vi "Measurement_Param_Global_Var.vi"() -> ()   [LabVIEW 2017]
panel:
  out "Sweep Parameters":T1
  in  "Average_en":bool
  out "ADC Cnfg Data":T2
  in  "Iterations":u16=13 caption="Iterations per Step" step=1
  in  "Settling time":u32=13 caption="Settling Time (ms)" max=4095 step=1
  in  "Vcm_2":dbl caption="Vcm ADC_2 (V)" min=0.0 max=3.3 step=0.001 format="%#.3f"
  in  "Vcm_1":dbl caption="Vcm ADC_1 (V)" min=0.0 max=3.3 step=0.001 format="%#.3f"
  in  "Sweep Vref2":bool caption="Sweep"
  in  "Nb of steps Vref2":u16 caption="Nb of steps" max=4095 step=1
  in  "Step size Vref2":u16 caption="Step size" max=4095 step=1
  in  "ADC Vref2":u16 caption="Start Value" max=4095 step=1
  in  "Sweep Vref1":bool caption="Sweep"
  in  "Sweep Vin":bool caption="Sweep"
  in  "Nb of steps Vref1":u16 caption="Nb of steps" max=4095 step=1
  in  "Step size Vref1":u16 caption="Step size" max=4095 step=1
  in  "ADC Vref1":u16 caption="Start Value" max=4095 step=1
  in  "Nb of steps Vin":u16 caption="Nb of steps" step=1
  in  "Step size Vin":u16 caption="Step size" step=1
  in  "ADC Vin":u16 caption="Start Value" step=1
  # "ADC Vin"
  # "Vref ADC_1"
  # "Vref ADC_2"
  # "Vcm"
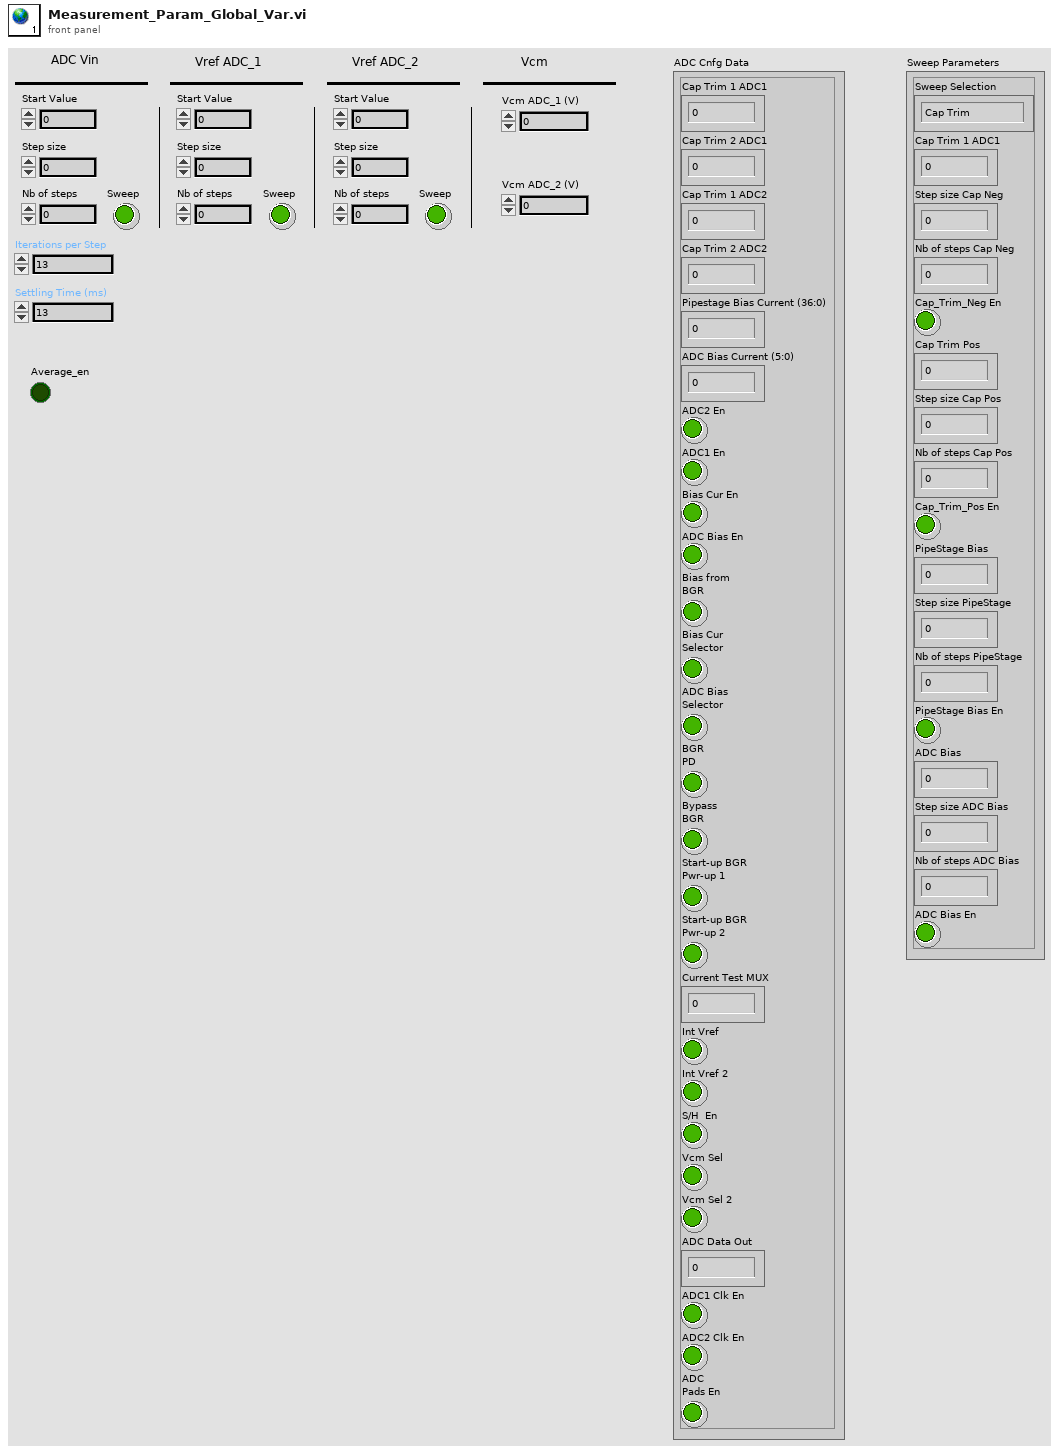
[diagram p1: front panel]
types:
  T1 = cluster{"Sweep Selection":enum32{"Cap Trim", "Bias Current", "Vreference"}, "Cap Trim 1 ADC1":u16, "Step size Cap Neg":u16, "Nb of steps Cap Neg":u16, "Cap_Trim_Neg En":bool, "Cap Trim Pos":u16, "Step size Cap Pos":u16, "Nb of steps Cap Pos":u16, "Cap_Trim_Pos En":bool, "PipeStage Bias":u64, "Step size PipeStage":u16, "Nb of steps PipeStage":u64, "PipeStage Bias En":bool, "ADC Bias":u8, "Step size ADC Bias":u16, "Nb of steps ADC Bias":u8, "ADC Bias En":bool}
  T2 = cluster{"Cap Trim 1 ADC1":u16, "Cap Trim 2 ADC1":u16, "Cap Trim 1 ADC2":u16, "Cap Trim 2 ADC2":u16, "Pipestage Bias Current (36:0)":u64, "ADC Bias Current (5:0)":u8, "ADC2 En":bool, "ADC1 En":bool, "Bias Cur En":bool, "ADC Bias En":bool, "Bias from\nBGR":bool, "Bias Cur\nSelector":bool, "ADC Bias\nSelector":bool, "BGR \nPD":bool, "Bypass\nBGR":bool, "Start-up BGR\nPwr-up 1":bool, "Start-up BGR\nPwr-up 2":bool, "Current Test MUX":u8, "Int Vref":bool, "Int Vref 2":bool, "S/H  En":bool, "Vcm Sel":bool, "Vcm Sel 2":bool, "ADC Data Out":u8, "ADC1 Clk En":bool, "ADC2 Clk En":bool, "ADC \nPads En":bool}
diagram:
